vi "Read Waveforms from Buffer.vi"(8 "error in (no error)":errorcluster, 11 "Waveforms (N Ch) in":refnum<class "Waveforms (N Ch).lvclass">) -> (0 "error out":errorcluster, 2 "waveforms":waveform(dbl)[](array[waveform]), 3 "Waveforms (N Ch) out":refnum<class "Waveforms (N Ch).lvclass">)   [LabVIEW 2017, in "Waveforms (N Ch).lvclass"]
uses:
  <vilib>/addons/_NISVFA/_Shared subVIs/Data Objects/Waveforms (DBL)/Waveforms (N Ch).lvclass
  <vilib>/addons/_NISVFA/_Shared subVIs/Data Objects/Waveforms (DBL)/Waveforms (N Ch).lvclass/Waveforms (N Ch).ctl
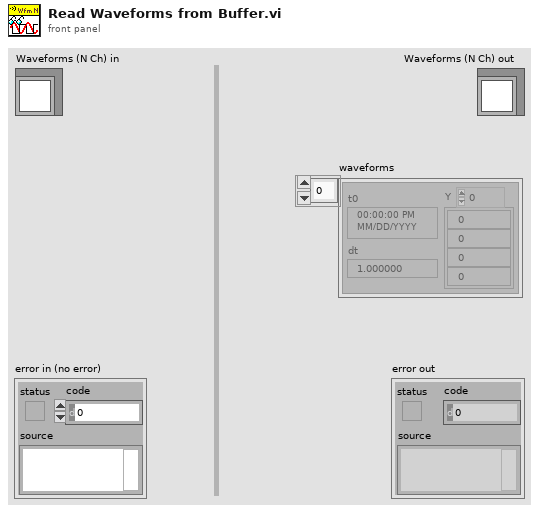
[diagram p1: front panel]
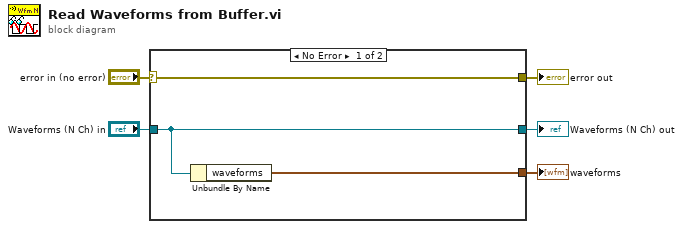
[diagram p0: block diagram]
diagram:
  n1 = case shown="No Error" "error in (no error)" {
    selector: "error in (no error)" -> [w8 w9]
    tunnel: [w8 w9] -> w4
    tunnel: [w6 w10] -> w2
    tunnel: "Waveforms (N Ch) in" -> [w6 w10]
    tunnel: [w7 _] -> w1
    frame No Error {
      n2 = Unbundle By Name(w6) -> ("waveforms"=w7:waveform(dbl)[])
    }
    frame Error {
    }
  }
  "error out" <- w4
  "Waveforms (N Ch) out" <- w2
  "waveforms" <- w1
